vi "StringArrayToTabDelimiter.vi"(10 "StringArray":string[](array[string])) -> (2 "String":string)   [LabVIEW 2015]
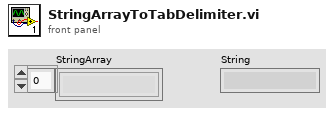
[diagram p1: front panel]
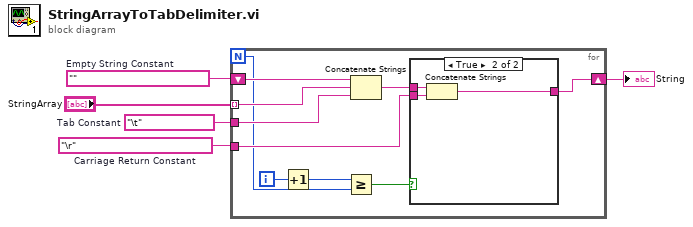
[diagram p0: block diagram]
diagram:
  w5 = ""  # Empty String Constant
  w3 = "\r"  # Carriage Return Constant
  w4 = "\t"  # Tab Constant
  n1 = for {
    N -> [w6]
    tunnel: "StringArray" -> [w14] mode=indexing
    shift-right: [w8] -> w2
    shift-left: w5 -> [w15]
    tunnel: w4 -> [w13]
    tunnel: w3 -> [w7]
    i -> [w12]
    n2 = Increment(x=w12) -> (x+1=w11:i32)
    n3 = Greater Or Equal?(x=w11, y=w6) -> (x >= y?=w10:bool)
    n4 = Concatenate Strings "Concatenate Strings"(w15, w14, w13) -> (w9:string)
    n5 = case shown="True" w10 {
      tunnel: w9 -> [w16 w19]
      tunnel: [w16 w18] -> w8
      tunnel: w7 -> [_ w17]
      frame False {
      }
      frame True {
        n6 = Concatenate Strings "Concatenate Strings"(w19, w17) -> (w18:string)
      }
    }
  }
  "String" <- w2
